vi "Load Stored Install Data.vi"(11 "Stored Install Data":path) -> (2 "Installed Files":path[](array[path]), 3 "Package Display Name":string)   [LabVIEW 2011, in "LVH-Toolbox.lvlib" / "Installer Tools.lvlib"]
uses:
  Installer Tools.lvlib
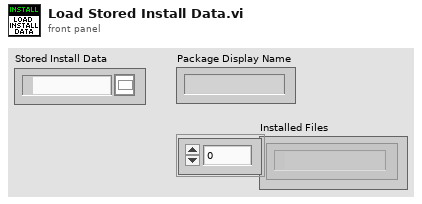
[diagram p1: front panel]
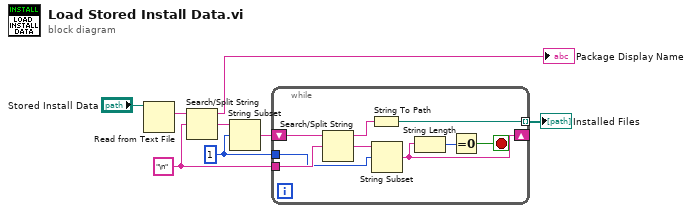
[diagram p0: block diagram]
diagram:
  w1 = 1 ("offset (0)")
  w2 = "\n" ("substring before match")
  n1 = Read from Text File(file (use dialog)="Stored Install Data") -> (text=w4:string)  [unwired: 3 in, 3 out]
  n2 = Search/Split String(string=w4, search string/char (-)=w2) -> (substring before match=→"Package Display Name":string, match + rest of string=w5:string)  [unwired: 1 in, 1 out]
  n3 = String Subset(string=w5, offset (0)=w1) -> (substring=w6:string)  [unwired: 1 in]
  n4 = while {
    shift-right: [w13] -> _
    shift-left: w6 -> [w16]
    tunnel: [w12] -> w8 mode=indexing
    tunnel: w2 -> [w11]
    tunnel: w1 -> [w10]
    stop <- w15 stop-if-true
    n5 = Search/Split String(string=w16, search string/char (-)=w11) -> (substring before match=w9:string, match + rest of string=w17:string)  [unwired: 1 in, 1 out]
    n6 = String To Path(string=w9) -> (path=w12:path)
    n7 = String Subset(string=w17, offset (0)=w10) -> (substring=w13:string)  [unwired: 1 in]
    n8 = String Length(string=w13) -> (length=w14:i32)
    n9 = Equal To 0?(x=w14) -> (x = 0?=w15:bool)
  }
  "Installed Files" <- w8
